vi "Msg.vi"(7 "Actor in":refnum<class "Actor.lvclass">, 11 "Create Msg in":refnum<class "Create Msg.lvclass">) -> (0 "error out":errorcluster, 2 "Destroy Self?":bool, 5 "Actor out":refnum<class "Actor.lvclass">)   [LabVIEW 2021, in "Create.lvlib" / "Create Msg.lvclass"]
uses:
  Create Msg.lvclass
  AAM/Actor/Actor.lvclass
  Create/Create.lvclass
  Create Msg.lvclass/Create Msg.ctl
  a4047ede-157f-4480-950e-247ce5526756.vi
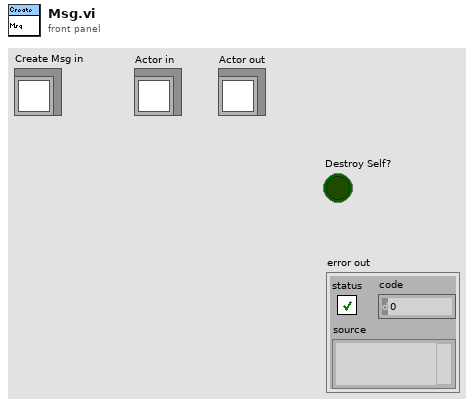
[diagram p1: front panel]
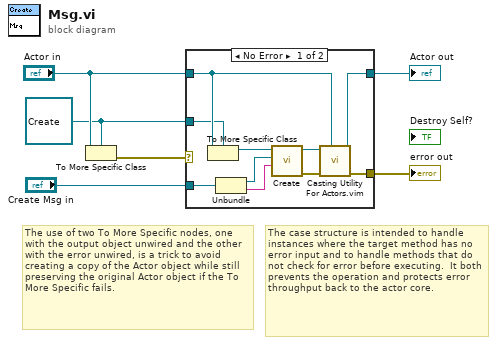
[diagram p0: block diagram]
diagram:
  w1 = refnum<class "Create.lvclass"> refnum ("Create.lvlib:Create.lvclass")
  # "The use of two To More Specific nodes, one with the output object unwired and the other with the error unwired, is a trick to avoid creating a copy of the Actor object while still preserving the original Actor object if the To More Specific fails."
  # "The case structure is intended to handle instances where the target method has no error input and to handle methods that do not check for error before executing.  It both prevents the operation and protects error throughput back to the actor core."
  n1 = To More Specific Class(target class=w1, reference="Actor in") -> (error out=w6:errorcluster)  [unwired: 1 in, 1 out]
  n2 = case shown="No Error" w6 {
    selector: w6 -> [_ w18]
    tunnel: [w14 w18] -> w4
    tunnel: [w15 w17] -> w2
    tunnel: "Actor in" -> [w16 w17]
    tunnel: w1 -> [w7 _]
    tunnel: "Create Msg in" -> [w13 _]
    frame No Error {
      n3 = To More Specific Class(target class=w7, reference=w16) -> (specific class reference=w12:refnum<class "Create.lvclass">)  [unwired: 1 in, 1 out]
      n4 = Unbundle(w13) -> (w8:refnum<class "Actor.lvclass">, w9:string)
      n5 = call-dynamic "Create.vi"("Alias"=w9, "Actor"=w8, "Create in"=w12) -> ("error out"=w10:errorcluster, "Create out"=w11:refnum<class "Create.lvclass">)  [unwired: 7 in]
      n6 = call "Casting Utility For Actors.vim"("type"=w16, "error in (no error)"=w10, "Actor in"=w11) -> ("error out"=w14:errorcluster, "Actor out"=w15:refnum<class "Actor.lvclass">)  [unwired: 7 in]
    }
    frame Error {
      # "If type check fails, pass the original object out again."
    }
  }
  "error out" <- w4
  "Actor out" <- w2
